vi "Escape String Literals for Query.vi"(9 "String":string, 11 "string-literal delimiter (')":string="'") -> (10 "escaped String":string)   [LabVIEW 2011]
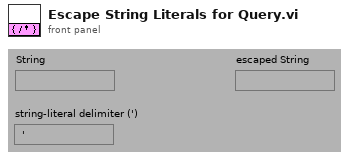
[diagram p1: front panel]
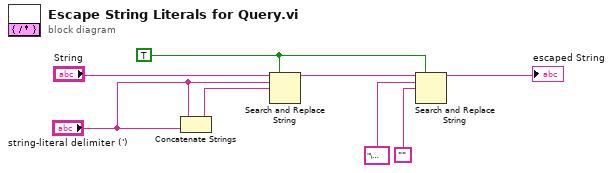
[diagram p0: block diagram]
diagram:
  w1 = TRUE
  n1 = Concatenate Strings("string-literal delimiter (')", "string-literal delimiter (')") -> (w6:string)
  n2 = Search and Replace String(replace all?=w1, input string="String", search string="string-literal delimiter (')", replace string=w6) -> (result string=w5:string)  [unwired: 1 in, 6 out]
  n3 = Search and Replace String(replace all?=w1, input string=w5, search string="\u0000", replace string="") -> (result string=→"escaped String":string)  [unwired: 1 in, 6 out]
